vi "Read_Waveform.vi"(8 "Error_In":errorcluster, 11 "I2C_In":refnum<class "I2C.lvclass">) -> (0 "Error_Out":errorcluster, 2 "I2C_Waveform":waveform(dbl)[](graph), 3 "I2C_Out":refnum<class "I2C.lvclass">)   [LabVIEW 2021, in "I2C.lvclass"]
doc: "Used to Read the I2C Waveform"
uses:
  I2C.lvclass
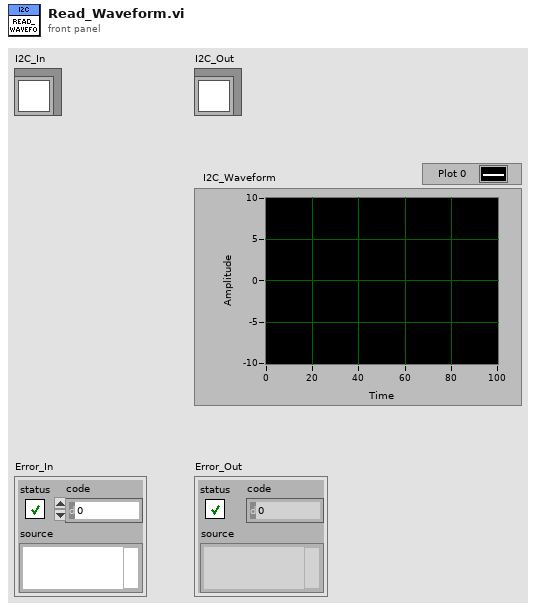
[diagram p1: front panel]
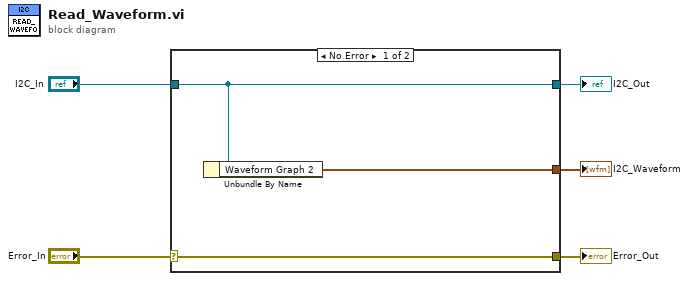
[diagram p0: block diagram]
diagram:
  n1 = case shown="No Error" "Error_In" {
    selector: "Error_In" -> [w8 w9]
    tunnel: [w8 w9] -> w4
    tunnel: [w7 w10] -> w2
    tunnel: "I2C_In" -> [w7 w10]
    tunnel: [w6 _] -> w1
    frame No Error {
      n2 = Unbundle By Name(w7) -> ("Waveform Graph 2"=w6:waveform(dbl)[])
    }
    frame Error {
    }
  }
  "Error_Out" <- w4
  "I2C_Out" <- w2
  "I2C_Waveform" <- w1
